vi "Servo (SubVI).vi"(6 "Center pixel in":dbl format="%#_13g", 9 "Pixel value in":dbl format="%#_13g", 10 "Position":dbl format="%#_13g", 11 "null offset":bool) -> (0 "Position 2":dbl, 1 "freq [Hz]":dbl=50.0, 2 "offset [%FS]":dbl, 3 "Duty":dbl)   [LabVIEW 2018]
uses:
  <vilib>/addons/control/pid/NI_PID_pid.lvlib
  <vilib>/addons/control/pid/pid.llb/PID (DBL).vi
panel:
  in  "Center pixel":dbl format="%#_13g"
  in  "Pixel value":dbl format="%#_13g"
  in  "Position.":dbl format="%#_13g"
  in  "PID gains":T1={"proportional gain (Kc)"=1.0, "integral time (Ti, min)"=0.01, "derivative time (Td, min)"=0.0} {"derivative time (Td, min)" format="%.3f"; "integral time (Ti, min)" format="%.4f"; "proportional gain (Kc)" format="%.3f"}
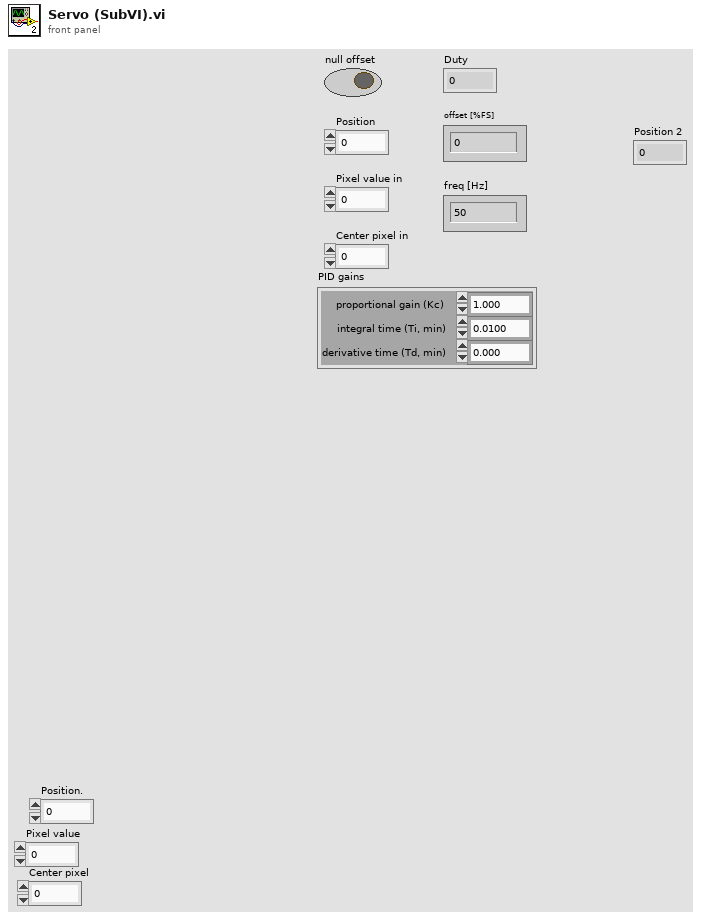
[diagram p1: front panel]
types:
  T1 = cluster{"proportional gain (Kc)":dbl, "integral time (Ti, min)":dbl, "derivative time (Td, min)":dbl}
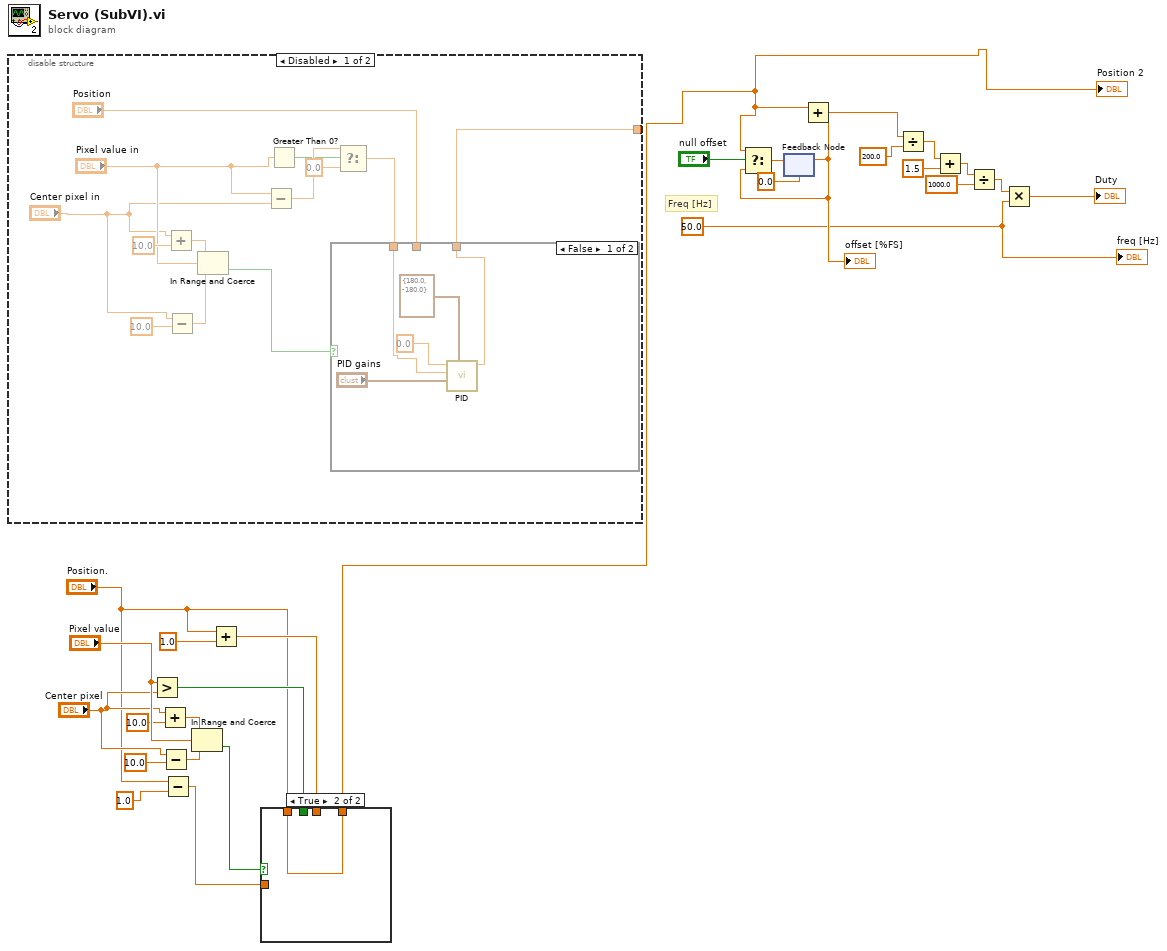
[diagram p0: block diagram]
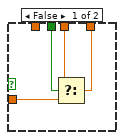
[diagram p2: hidden frame]
diagram:
  w20 = 50.0 ("freq [Hz]")
  # "Freq [Hz]"
  n1 = disable-structure shown="Disabled" {
    disable-tunnel: [w34 _] -> _
    frame Disabled {
      n2 = Add(x="Center pixel in", y=10.0) -> (x+y=w39:dbl)
      n3 = Subtract(x="Center pixel in", y=10.0) -> (x-y=w37:dbl)
      n4 = In Range and Coerce(upper limit=w39, x="Pixel value in", lower limit=w37) -> (In Range?=w36:bool)  [unwired: 1 out]
      n5 = Subtract(x="Pixel value in", y="Center pixel in") -> (x-y=w32:dbl)
      n6 = Greater Than 0?(x="Pixel value in") -> (x > 0?=w31:bool)
      n7 = Select(t=w32, s=w31, f=0.0) -> (s? t:f=w33:dbl)
      n8 = case shown="False" w36 {
        tunnel: [w41 w46] -> w34
        tunnel: "Position" -> [_ w46]
        tunnel: w33 -> [w43 _]
        frame False {
          n9 = call-poly <vilib>:"PID.vi"("output range"=cluster{"output high":dbl, "output low":dbl} {"output high"=180.0, "output low"=-180.0}, "PID gains"="PID gains", "process variable"=w43, "setpoint"=0.0) -> ("output"=w41:dbl)  [unwired: 6 in, 1 out]
        }
        frame True {
        }
      }
    }
    frame Enabled {
    }
  }
  n10 = Greater?(x="Pixel value", y="Center pixel") -> (0:w4:bool)
  n11 = Add(x="Center pixel", y=10.0) -> (x+y=w10:dbl)
  n12 = Subtract(x="Center pixel", y=10.0) -> (x-y=w7:dbl)
  n13 = Subtract(x="Position.", y=1.0) -> (x-y=w5:dbl)
  n14 = In Range and Coerce(upper limit=w10, x="Pixel value", lower limit=w7) -> (In Range?=w6:bool)  [unwired: 1 out]
  n15 = Add(x="Position.", y=1.0) -> (x+y=w3:dbl)
  n16 = case shown="True" w6 {
    tunnel: w5 -> [w50 _]
    tunnel: w4 -> [w49 _]
    tunnel: w3 -> [w48 _]
    tunnel: [w47 w51] -> w1
    tunnel: "Position." -> [_ w51]
    frame False {
      n17 = Select(t=w48, s=w49, f=w50) -> (s? t:f=w47:dbl)
    }
    frame True {
    }
  }
  "Position 2" <- w1
  n18 = feedback #1(0.0 ("position [%FS]")) -> (w24:dbl)
  "offset [%FS]" <- w24
  n19 = Select(t=w1, s="null offset", f=w24) -> (s? t:f=w22:dbl)
  n20 = feedback-in #1(w22) -> ()
  n21 = Add(x=w1, y=w24) -> (x+y=w23:dbl)
  n22 = Divide(x=w23, y=200.0) -> (x/y=w16:dbl)
  n23 = Add(x=w16, y=1.5) -> (x+y=w18:dbl)
  n24 = Divide(x=w18, y=1000.0) -> (x/y=w25:dbl)
  n25 = Multiply(x=w25, y=w20) -> (x*y=→"Duty":dbl)
  "freq [Hz]" <- w20
